vi "runAO_img.vi"   [LabVIEW 2015]
uses:
  waveforms/usedAOindepofwf.vi
  Misc/add channel to active arrayv2.vi
  Objects/configuration.vi
  Objects/2pparameters.vi
types:
  T1 = cluster{"AO":refnum<k21>[], "E_AO":errorcluster[]}
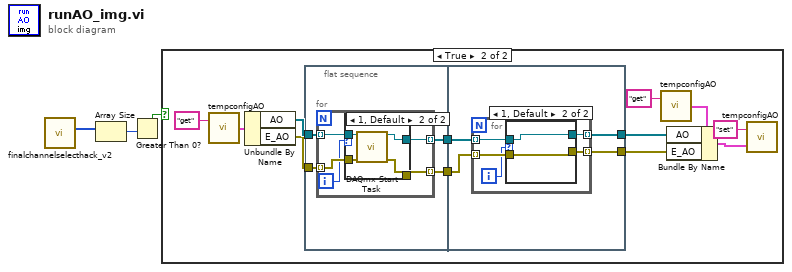
[diagram p0: block diagram]
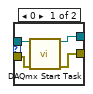
[diagram p4: hidden frame]
diagram:
  n1 = call "finalchannelselecthack_v2.vi"() -> ("devices"=w1:u32[])  [unwired: 1 in, 1 out]
  n2 = Array Size(array=w1) -> (size(s)=w3:i32)
  n3 = Greater Than 0?(x=w3) -> (x > 0?=w2:bool)
  n4 = case shown="True" w2 {
    frame False {
    }
    frame True {
      n5 = call "tempconfigAO.vi"("command"="get") -> ("Temp Config out"=w12:T1)  [unwired: 1 in]
      n6 = Unbundle By Name(w12) -> ("AO"=w9:refnum<k21>[], "E_AO"=w8:errorcluster[])
      n7 = flat-sequence {
        tunnel: w9 -> [w19]
        tunnel: w8 -> [w18]
        tunnel: [w17] -> w7
        tunnel: [w16] -> w6
        tunnel: w7 -> [w34]
        tunnel: w6 -> [w33]
        tunnel: [w32] -> w5
        tunnel: [w31] -> w4
        frame #0 {
          n8 = for {
            tunnel: w19 -> [w24] mode=indexing
            tunnel: [w21] -> w16 mode=indexing
            tunnel: w18 -> [w22] mode=indexing
            tunnel: [w23] -> w17 mode=indexing
            i -> [w20]
            n9 = case shown="1, Default" w20 {
              tunnel: w24 -> [w26 w30]
              tunnel: [w26 w29] -> w23
              tunnel: w22 -> [w25 w28]
              tunnel: [w25 w27] -> w21
              frame 0 {
              }
              frame 1, Default {
                n10 = call <vilib>:"DAQmx Start Task.vi"("task/channels in"=w30, "error in"=w28) -> ("task out"=w29:refnum<k21>, "error out"=w27:errorcluster)  [unwired: 12 in]
              }
            }
          }
        }
        frame #1 {
          n11 = for {
            tunnel: w34 -> [w39] mode=indexing
            tunnel: w33 -> [w38] mode=indexing
            tunnel: [w37] -> w32 mode=indexing
            tunnel: [w36] -> w31 mode=indexing
            i -> [w35]
            n12 = case shown="1, Default" w35 {
              tunnel: w39 -> [w43 w44]
              tunnel: w38 -> [w42 w45]
              tunnel: [w41 w44] -> w37
              tunnel: [w40 w45] -> w36
              frame 0 {
                n13 = call <vilib>:"DAQmx Start Task.vi"("task/channels in"=w43, "error in"=w42) -> ("task out"=w41:refnum<k21>, "error out"=w40:errorcluster)  [unwired: 12 in]
              }
              frame 1, Default {
              }
            }
          }
        }
      }
      n14 = call "tempconfigAO.vi"("command"="get") -> ("Temp Config out"=w11:T1)  [unwired: 1 in]
      n15 = Bundle By Name(cluster=w11, "AO"=w5, "E_AO"=w4) -> (w10:T1)
      n16 = call "tempconfigAO.vi"("Temp Config in"=w10, "command"="set") -> ()  [unwired: 1 out]
    }
  }
